vi "Controller Receive PS Manual Setpoints.vi"(0 "PS Setpoints FIFO":refnum<k33>, 2 "Number of Correctors":i32, 7 "FC PS Setpoints":sgl[](array[numeric]), 9 "FC PS Mode":u16, 11 "error in (no error)":errorcluster) -> (4 "Raw PS Setpoints + PS ON-OFF":dbl[](array[numeric]), 6 "PS Setpoints":dbl[](array[numeric]), 8 "PS ON-OFF (per PS Rack)":u8[](array[numeric]), 10 "new PS Setpoints?":bool, 15 "error out":errorcluster)   [LabVIEW 2011, in "Controller VIs.lvlib"]
uses:
  Controller VIs.lvlib
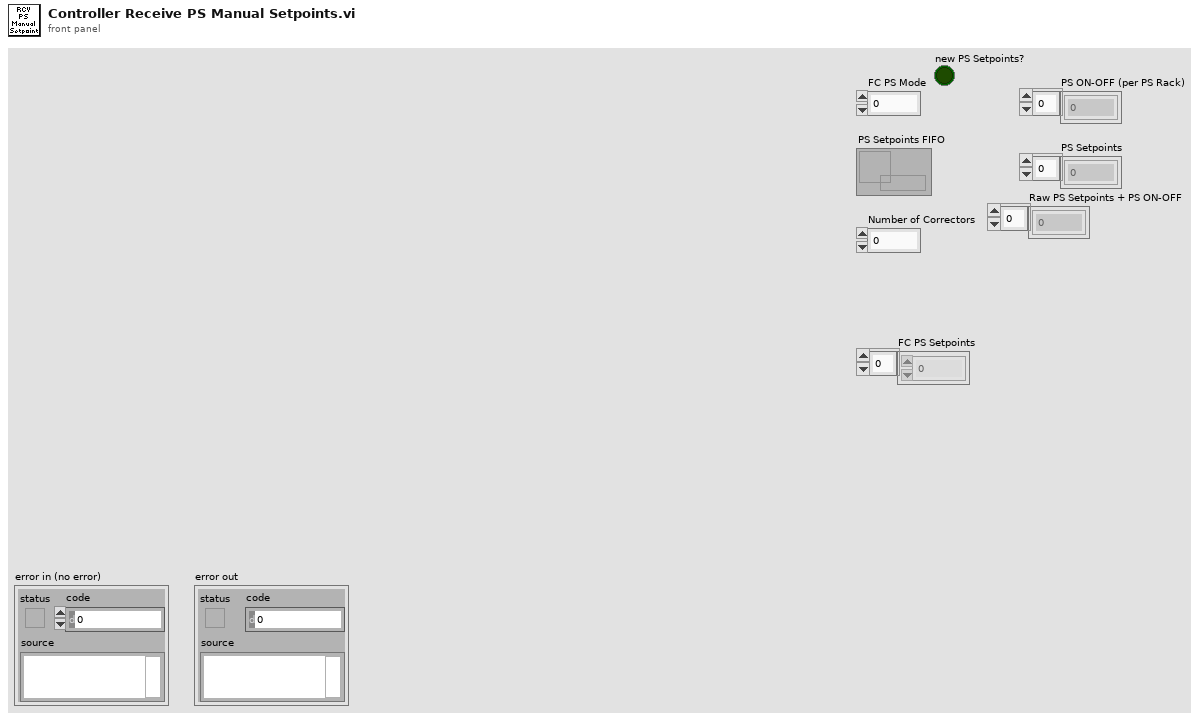
[diagram p1: front panel]
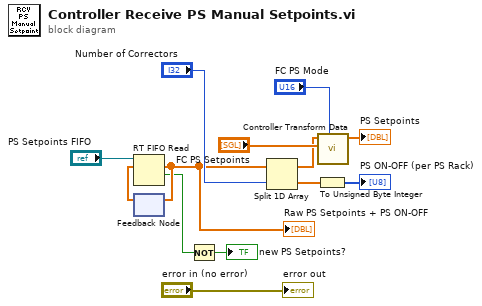
[diagram p0: block diagram]
diagram:
  n1 = feedback #1() -> (w3:dbl[])  [unwired: 1 in]
  n2 = RT FIFO Read(0:"PS Setpoints FIFO", 1:w3) -> (9:w4:dbl[], 10:w2:bool)  [unwired: 2 in, 3 out]
  "Raw PS Setpoints + PS ON-OFF" <- w4
  n3 = feedback-in #1(w4) -> ()
  n4 = Not(x=w2) -> (.not. x?=→"new PS Setpoints?":bool)
  n5 = Split 1D Array(array=w4, index="Number of Correctors") -> (first subarray=w6:dbl[], second subarray=w7:dbl[])
  n6 = To Unsigned Byte Integer(number=w7) -> (unsigned 8bit integer=→"PS ON-OFF (per PS Rack)":u8[])
  n7 = call "Controller Transform Data.vi"("Mode (Transparent)"="FC PS Mode", "New Data"="FC PS Setpoints", "Data"=w6) -> ("Transformed Data"=→"PS Setpoints":dbl[])  [unwired: 7 in, 1 out]
  "error out" <- "error in (no error)"
